vi "Check if configuration files exist.vi"(8 "error in (no error)":errorcluster, 11 "GalvoBase in":refnum<class "InVivo_ImagingModeSPIM.lvclass">) -> (0 "error out":errorcluster, 2 "configuration file exists?":bool, 3 "GalvoBase out":refnum<class "InVivo_ImagingModeSPIM.lvclass">)   [LabVIEW 2012, in "InVivo_ImagingModeSPIM.lvclass"]
doc: "Checks whether all required configuration files for the component exist."
uses:
  InVivo_ImagingModeSPIM.lvclass
  <vilib>/Distrio/Murmex/Murmex/Murmex.lvclass
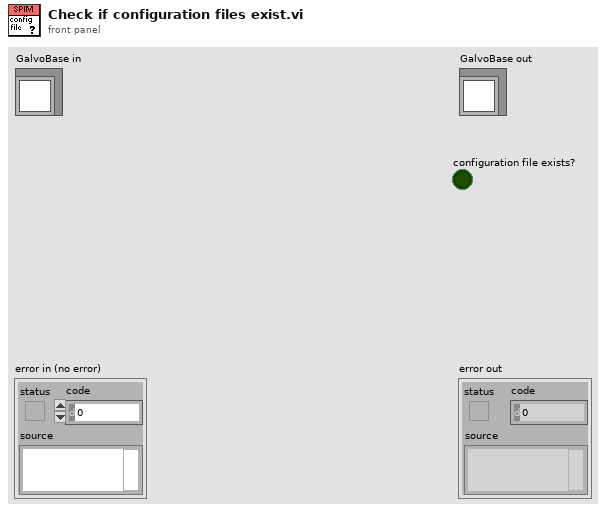
[diagram p1: front panel]
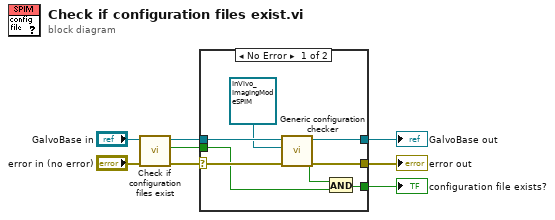
[diagram p0: block diagram]
diagram:
  n1 = call-parent "Check if configuration files exist.vi"("error in (no error)"="error in (no error)", "MurmexBase in"="GalvoBase in") -> ("error out"=w6:errorcluster, "configuration file exists?"=w1:bool, "MurmexBase out"=w4:refnum<class "InVivo_ImagingModeSPIM.lvclass">)  [unwired: 7 in]
  n2 = case shown="No Error" w6 {
    selector: w6 -> [w16 w17]
    tunnel: [w15 w17] -> w5
    tunnel: w4 -> [w14 w18]
    tunnel: [w13 w18] -> w3
    tunnel: [w10 _] -> w2
    tunnel: w1 -> [w9 _]
    frame No Error {
      n3 = call <vilib>:"Generic configuration checker.vi"("error in (no error)"=w16, "inheritance level"=refnum<class "InVivo_ImagingModeSPIM.lvclass"> refnum ("Galvo.lvclass"), "Murmex in"=w14) -> ("error out"=w15:errorcluster, "configuration file exists?"=w11:bool, "Murmex out"=w13:refnum<class "InVivo_ImagingModeSPIM.lvclass">)  [unwired: 6 in]
      n4 = And(x=w11, y=w9) -> (x .and. y?=w10:bool)
    }
    frame Error {
    }
  }
  "error out" <- w5
  "GalvoBase out" <- w3
  "configuration file exists?" <- w2
